vi "ARM angles.vi"() -> ()   [LabVIEW 2018]
panel:
  out "base busy":bool
  out "base sensor":bool
  out "gripper":i32
  out "base":i32
  out "wrist":i32
  out "elbow":i32
  out "shoulder":i32
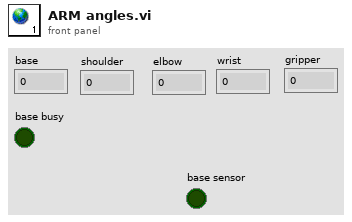
[diagram p1: front panel]
diagram:
